vi "cache.vi"(5 "target":string, 7 "project path":path, 9 "write (T): read (F)":bool, 10 "CCSymbols in":string) -> (2 "CCSymbols out":string)   [LabVIEW 2019, in "Conditional Disable Build Actions.lvlib"]
uses:
  <vilib>/Utility/config.llb/Write Key (String).vi
  <vilib>/Utility/config.llb/Read Key (String).vi
  Conditional Disable Build Actions.lvlib
  <vilib>/Utility/config.llb/NI_LVConfig.lvlib
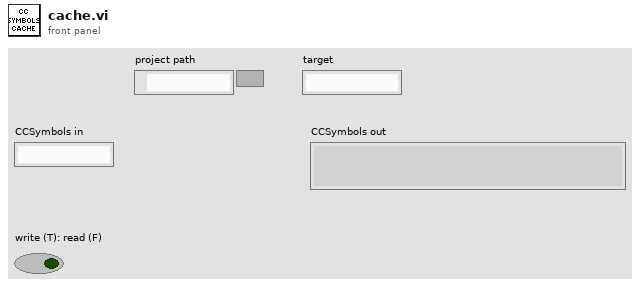
[diagram p1: front panel]
types:
  T1 = typedef "NI_LVConfig.lvlib/Config Data RefNum.ctl" = refnum<k1>
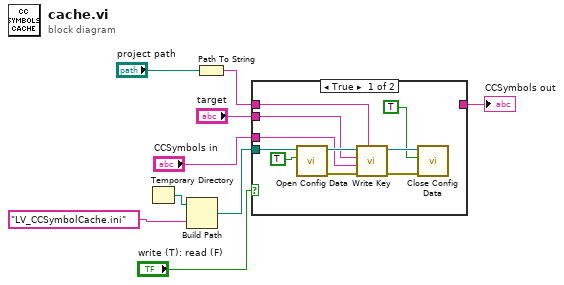
[diagram p0: block diagram]
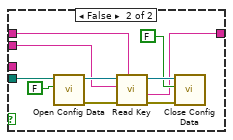
[diagram p2: hidden frame]
diagram:
  n1 = Temporary Directory() -> (w7:path)
  n2 = Build Path(base path=w7, name or relative path="LV_CCSymbolCache.ini") -> (appended path=w5:path)
  n3 = Path To String(path="project path") -> (string=w3:string)
  n4 = case shown="True" "write (T): read (F)" {
    tunnel: "CCSymbols in" -> [w13 _]
    tunnel: w5 -> [w19 w29]
    tunnel: w3 -> [w11 w21]
    tunnel: [_ w22] -> w2
    tunnel: "target" -> [w10 w20]
    frame True {
      n5 = call <vilib>:"Open Config Data.vi"("create file if necessary (T)"=TRUE, "configuration file path"=w19) -> ("error out"=w17:errorcluster, "refnum"=w16:T1)  [unwired: 7 in, 1 out]
      n6 = call-poly <vilib>:"Write Key.vi"("section"=w11, "error in (no error)"=w17, "value"=w13, "key"=w10, "refnum"=w16) -> ("error out"=w14:errorcluster, "refnum out"=w15:T1)  [unwired: 4 in, 1 out]
      n7 = call <vilib>:"Close Config Data.vi"("error in (no error)"=w14, "write file if changed (T)"=TRUE, "refnum"=w15) -> ()  [unwired: 7 in, 2 out]
    }
    frame False {
      n8 = call <vilib>:"Open Config Data.vi"("create file if necessary (T)"=FALSE, "configuration file path"=w29) -> ("error out"=w27:errorcluster, "refnum"=w26:T1)  [unwired: 7 in, 1 out]
      n9 = call-poly <vilib>:"Read Key.vi"("section"=w21, "error in (no error)"=w27, "key"=w20, "refnum"=w26) -> ("error out"=w24:errorcluster, "value"=w22:string, "refnum out"=w25:T1)  [unwired: 4 in, 1 out]
      n10 = call <vilib>:"Close Config Data.vi"("error in (no error)"=w24, "write file if changed (T)"=FALSE, "refnum"=w25) -> ()  [unwired: 7 in, 2 out]
    }
  }
  "CCSymbols out" <- w2
